vi "find_FlagObject_by_Name.vi"(10 "Flag Name":string, 11 "FlagObj Array":refnum<class "flag.lvclass">[](array[class])) -> (0 "index of Object in Array":i32, 1 "found?":bool, 2 "found FlagObj out":refnum<class "flag.lvclass">, 3 "FlagObj Array out":refnum<class "flag.lvclass">[](array[class]))   [LabVIEW 2018]
doc: "Find the correct FlagObject by the Name of the Flag"
uses:
  Classes/Flags/flag.lvclass
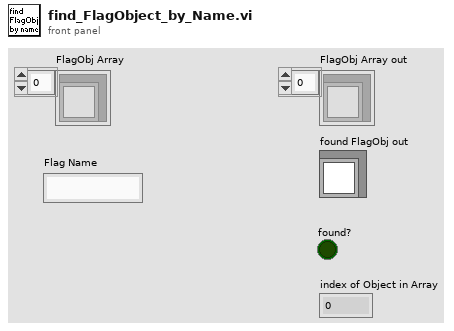
[diagram p1: front panel]
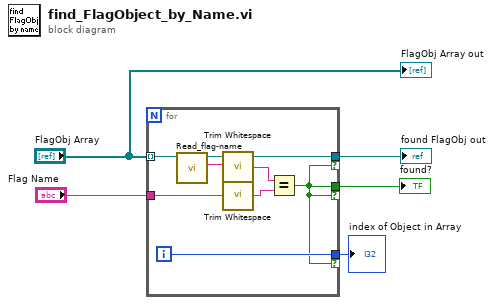
[diagram p0: block diagram]
diagram:
  n1 = for {
    tunnel: "Flag Name" -> [w13]
    tunnel: [w10] -> w4 if=w6
    tunnel: "FlagObj Array" -> [w8] mode=indexing
    tunnel: [w6] -> w3 if=w6
    tunnel: [w7] -> w1 if=w6
    i -> [w7]
    n2 = call-dynamic "Read_flag-name.vi"("flag in"=w8) -> ("flag name"=w9:string, "flag out"=w10:refnum<class "flag.lvclass">)  [unwired: 8 in, 1 out]
    n3 = call <vilib>:"Trim Whitespace.vi"("string"=w9) -> ("trimmed string"=w12:string)  [unwired: 1 in]
    n4 = call <vilib>:"Trim Whitespace.vi"("string"=w13) -> ("trimmed string"=w11:string)  [unwired: 1 in]
    n5 = Equal?(x=w12, y=w11) -> (x = y?=w6:bool)
  }
  "found FlagObj out" <- w4
  "found?" <- w3
  "index of Object in Array" <- w1
  "FlagObj Array out" <- "FlagObj Array"
